vi "GPIB_Server.vi"(4 "Case":T1, 5 "byte count":i32, 6 "error in":errorcluster, 7 "mode (0)":i16, 8 "timeout ms (488.2 global)":i32, 9 "data In":string, 10 "address string":string) -> (0 "error out":errorcluster, 2 "status":bool[](array[boolean]), 3 "data Out":string)   [LabVIEW 2010]
uses:
  Controls/GPIB_Mode.ctl
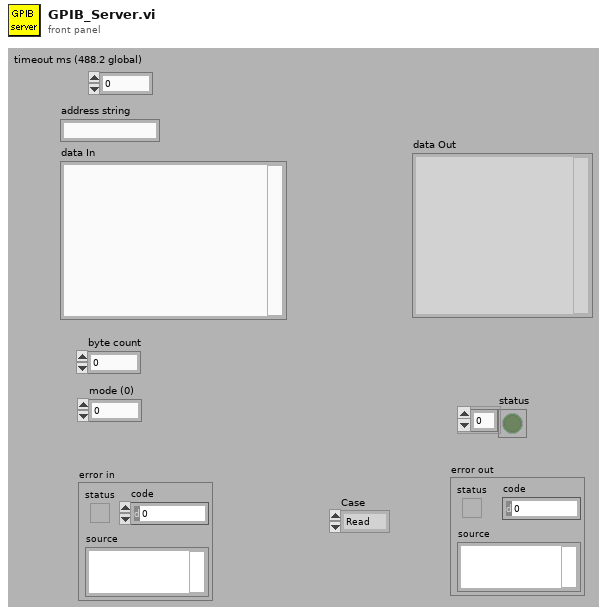
[diagram p1: front panel]
types:
  T1 = typedef "GPIB_Mode.ctl" = enum16{"Read", "Write", "Trigger", "Poll"}
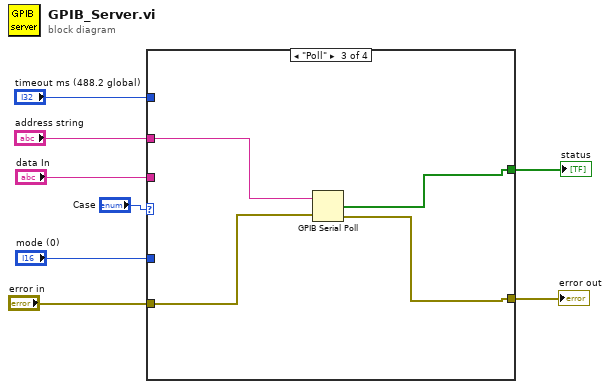
[diagram p0: block diagram]
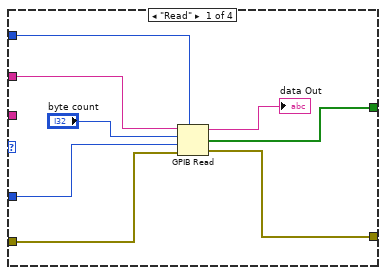
[diagram p2: hidden frame]
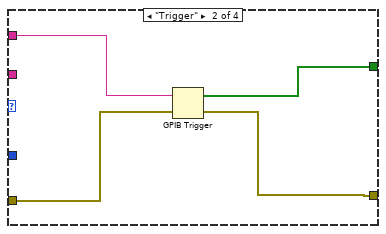
[diagram p3: hidden frame]
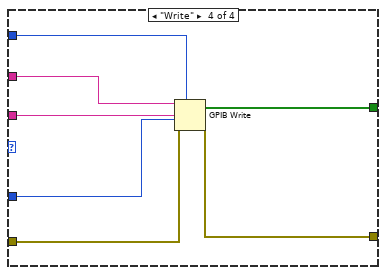
[diagram p4: hidden frame]
diagram:
  n1 = case shown="\"Poll\"" "Case" {
    tunnel: "address string" -> [w15 w20 w22 w31]
    tunnel: "data In" -> [_ _ _ w30]
    tunnel: "mode (0)" -> [w13 _ _ w29]
    tunnel: "error in" -> [w12 w19 w24 w28]
    tunnel: [w11 w18 w23 w27] -> w4
    tunnel: [w10 w17 w21 w26] -> w3
    tunnel: "timeout ms (488.2 global)" -> [w16 _ _ w25]
    frame "Read" {
      n2 = GPIB Read(0:w15, 1:"byte count", 2:w13, 3:w12, 4:w16) -> (5:→"data Out":string, 6:w10:bool[], 7:w11:errorcluster)
    }
    frame "Trigger" {
      n3 = GPIB Trigger(2:w19, 3:w20) -> (0:w18:errorcluster, 1:w17:bool[])
    }
    frame "Poll" {
      n4 = GPIB Serial Poll(0:w22, 1:w24) -> (3:w21:bool[], 4:w23:errorcluster)  [unwired: 1 out]
    }
    frame "Write" {
      n5 = GPIB Write(0:w31, 1:w30, 2:w29, 3:w28, 4:w25) -> (5:w26:bool[], 6:w27:errorcluster)
    }
  }
  "error out" <- w4
  "status" <- w3
